vi "main.vi"() -> ()   [LabVIEW 2023]
panel:
  out "On/Off Light":bool
  in  "On/Off":bool
  out "Hours":i16
  out "Minutes":i16
  out "Seconds":i16
  in  "Stop":bool
  out "Waveform Chart - Temperatures":T1(graph)
  out "Waveform Chart - Control Signal":dbl[](graph)
  out "Temp [C]":dbl=29.659641078261295
  out "Error Term":dbl
  in  "Tab Control":T2(tab)=enum."Air heater model parameters"
  in  "Location of Sensor":string="Stue"
  out "Start seconds":dbl
  out "Logging seconds":dbl
  in  "MA Filter":bool=TRUE
  out "Control Signal [V]":dbl format="%#_2g"
  in  "Desired Temperature [deg C]":dbl(slide)=30.0 scale=20.0..40.0
  in  "Time Step [s]":dbl=0.1
  in  "Air Heater Params":T3={"Temp_init [C]"=22.0, "K [C/V]"=3.2, "theta_t [s]"=5.5, "theta_d [s]"=3.0, "theta_d_out_init [V]"=0.0, "theta_d_max [s]"=5.0}
  in  "Temp Environment [C]":dbl(slide)=22.0 scale=0.0..35.0
  # "Program Runtime:"
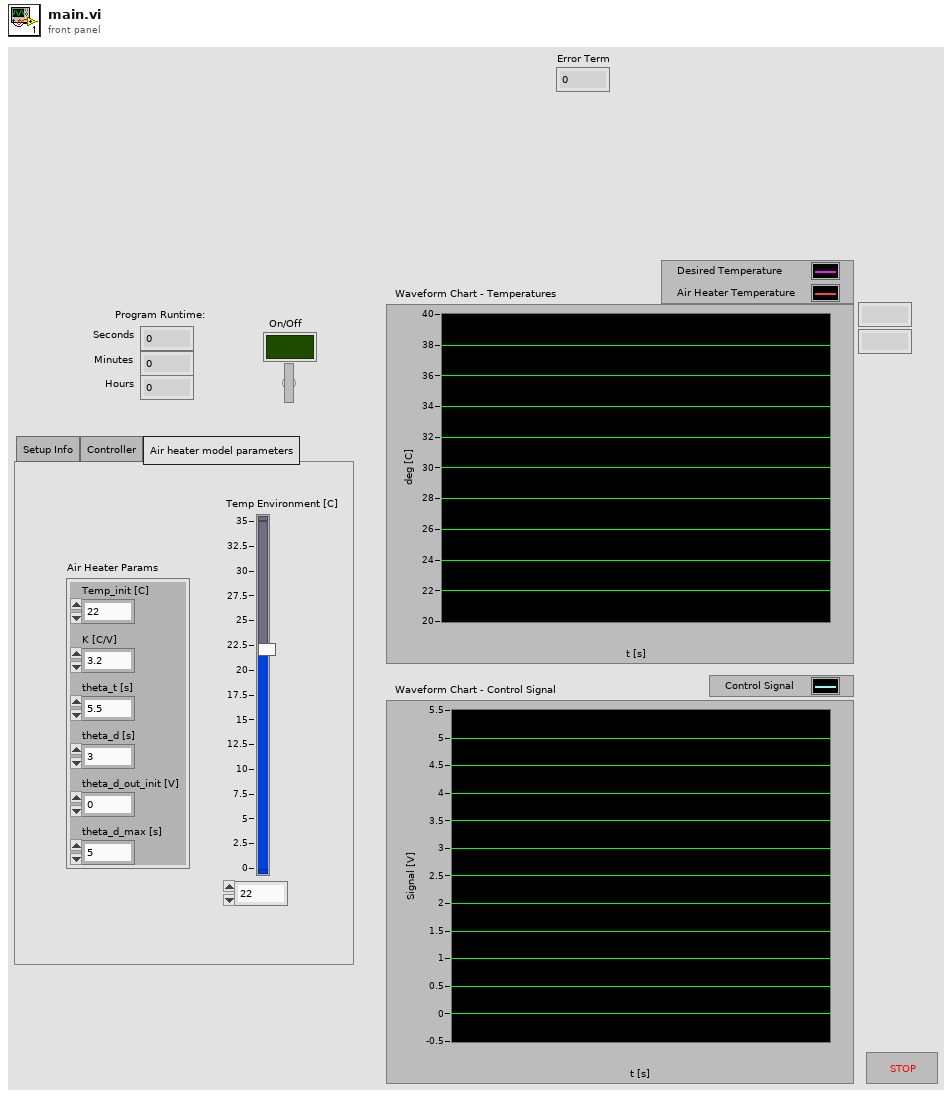
[diagram p1: front panel]
types:
  T1 = cluster{"Desired Temperature [deg C]":dbl, "Temp [C]":dbl}
  T2 = enum32{"Setup Info", "Controller", "Air heater model parameters"}
  T3 = cluster{"Temp_init [C]":dbl, "K [C/V]":dbl, "theta_t [s]":dbl, "theta_d [s]":dbl, "theta_d_out_init [V]":dbl, "theta_d_max [s]":dbl}
  T4 = cluster{"Desired Temperature [deg C]":dbl, "Temp [C]":dbl}[]
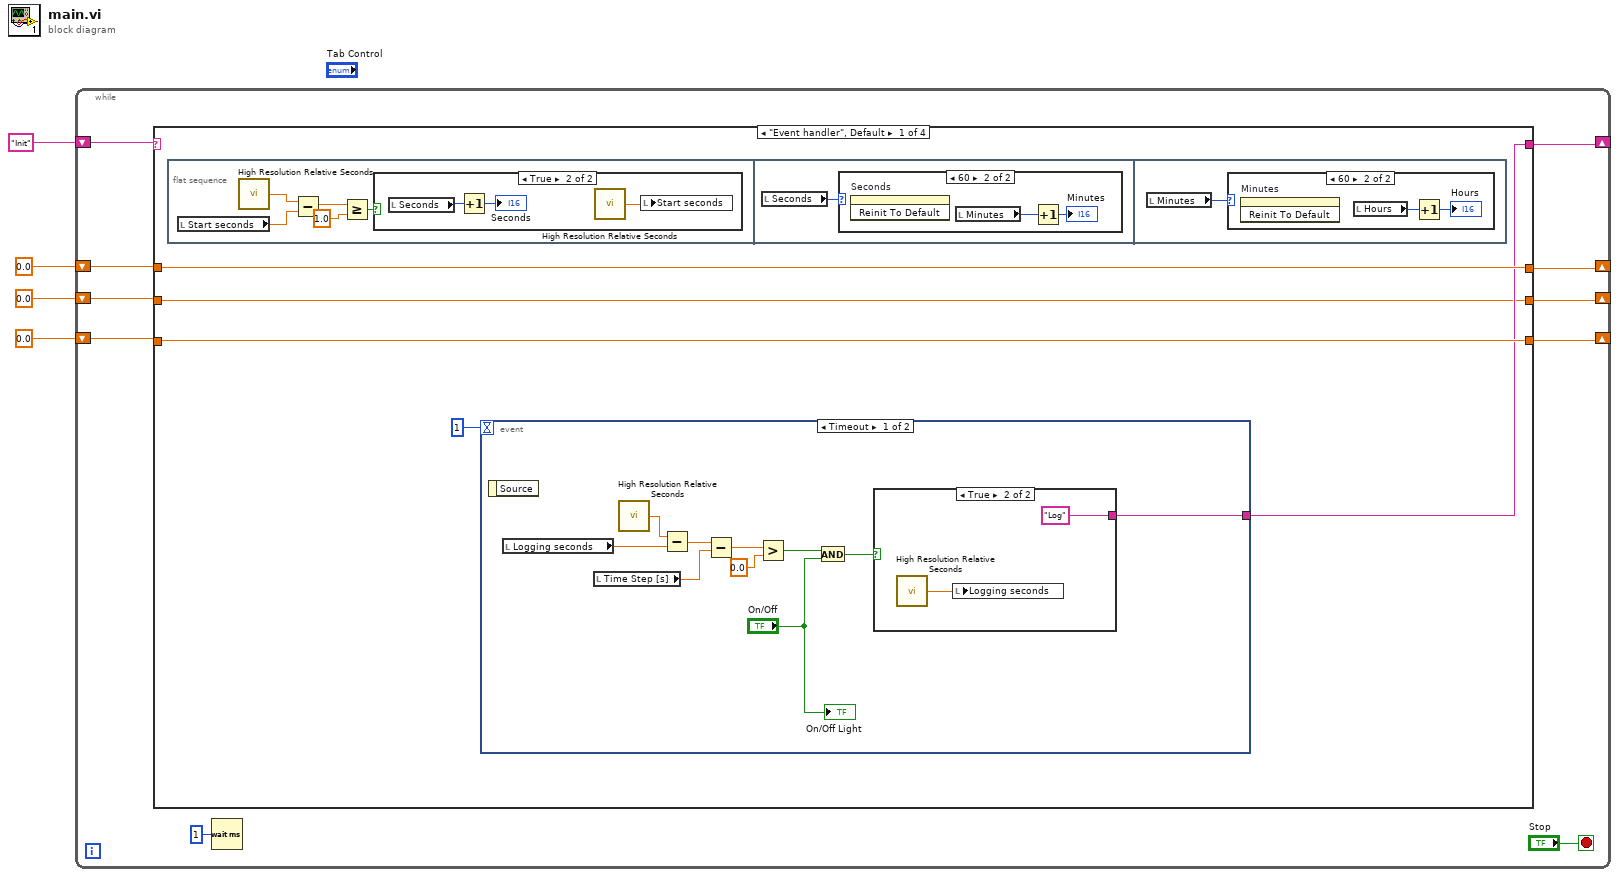
[diagram p0: block diagram]
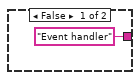
[diagram p2: hidden frame]
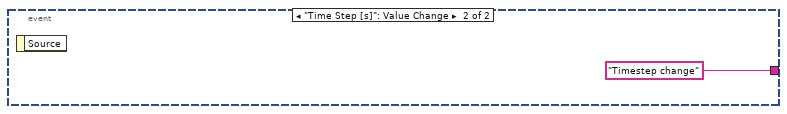
[diagram p3: hidden frame]
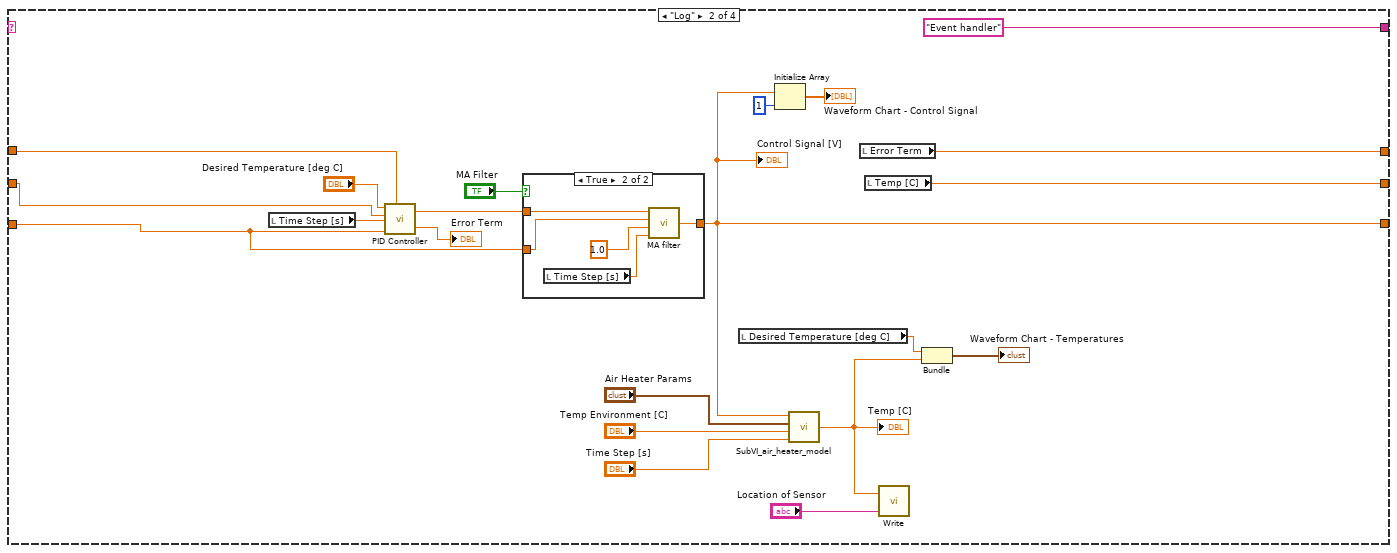
[diagram p7: hidden frame]
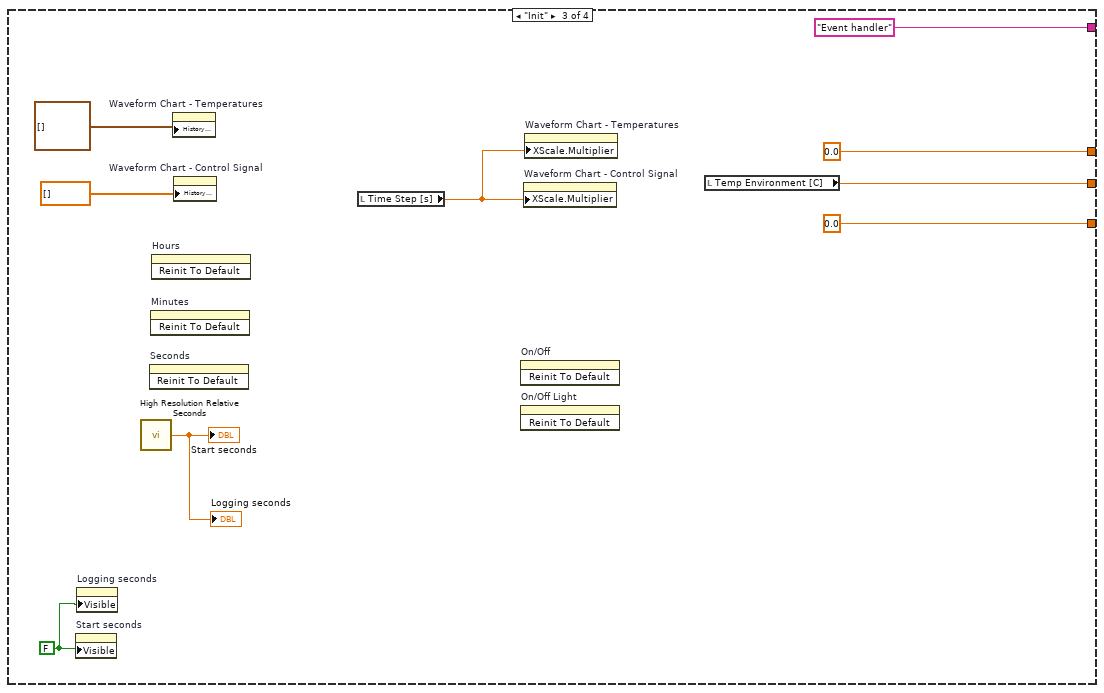
[diagram p9: hidden frame]
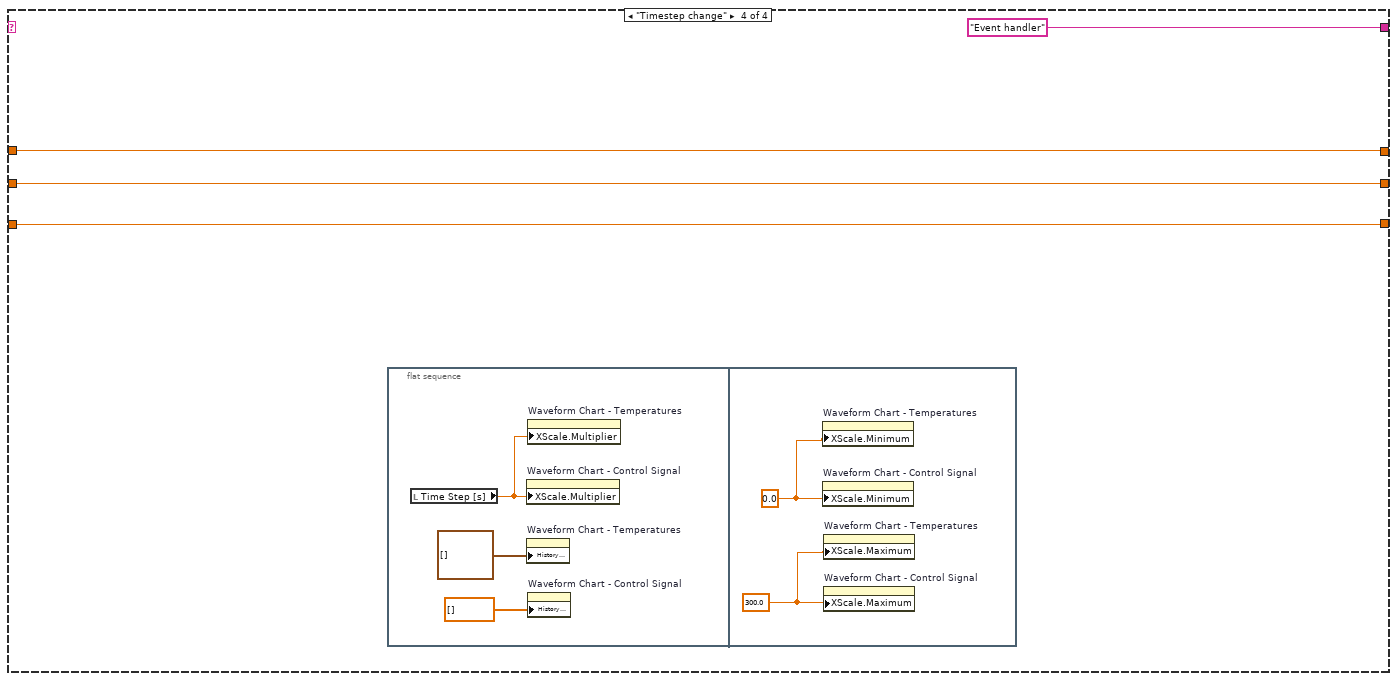
[diagram p10: hidden frame]
diagram:
  n1 = while {
    shift-right: [w8] -> _
    shift-left: "Init" -> [w13]
    shift-right: [w7] -> _
    shift-left: 0.0 ("yf") -> [w11]
    shift-right: [w6] -> _
    shift-left: 0.0 ("Error Term") -> [w10]
    shift-right: [w5] -> _
    shift-left: 0.0 ("Temp Environment [C]") -> [w9]
    stop <- "Stop" stop-if-true
    n2 = case shown="\"Event handler\", Default" w13 {
      tunnel: [w17 "Event handler" "Event handler" "Event handler"] -> w8
      tunnel: [w19 w52 0.0 ("yf") w87] -> w7
      tunnel: w11 -> [w19 w56 _ w87]
      tunnel: w10 -> [w18 w58 _ w86]
      tunnel: [w18 w57 0.0 ("Error Term") w86] -> w6
      tunnel: [w15 w55 w78 w84] -> w5
      tunnel: w9 -> [w15 w50 _ w84]
      frame "Event handler", Default {
        n3 = flat-sequence {
          frame #0 {
            n4 = local read "Start seconds"() -> (w37:dbl)
            n5 = call <vilib>:"High Resolution Relative Seconds.vi"() -> ("relative seconds"=w38:dbl)
            n6 = Subtract(x=w38, y=w37) -> (x-y=w36:dbl)
            n7 = Greater Or Equal?(x=w36, y=1.0) -> (x >= y?=w34:bool)
            n8 = case shown="True" w34 {
              frame False {
              }
              frame True {
                n9 = local read "Seconds"() -> (w39:i16)
                n10 = Increment(x=w39) -> (x+1=→"Seconds":i16)
                n11 = call <vilib>:"High Resolution Relative Seconds.vi"() -> ("relative seconds"=w41:dbl)
                n12 = local write "Start seconds"(w41) -> ()
              }
            }
          }
          frame #1 {
            n13 = local read "Seconds"() -> (w42:i16)
            n14 = case shown="60" w42 {
              frame 0, Default {
              }
              frame 60 {
                n15 = invoke on="Seconds" class="DigNum (strict)" method="Reinit To Default"() -> ()  [unwired: 3 in, 3 out]
                n16 = local read "Minutes"() -> (w43:i16)
                n17 = Increment(x=w43) -> (x+1=→"Minutes":i16)
              }
            }
          }
          frame #2 {
            n18 = local read "Minutes"() -> (w45:i16)
            n19 = case shown="60" w45 {
              frame 0, Default {
              }
              frame 60 {
                n20 = invoke on="Minutes" class="DigNum (strict)" method="Reinit To Default"() -> ()  [unwired: 3 in, 3 out]
                n21 = local read "Hours"() -> (w47:i16)
                n22 = Increment(x=w47) -> (x+1=→"Hours":i16)
              }
            }
          }
        }
        n23 = event shown="[0] Timeout" {
          selector: _ -> [_ _]
          dyn-events: _ -> [_ _]
          timeout: 1 -> [_ _]
          tunnel: [w25 "Timestep change"] -> w17
          event Timeout {
            n24 = event-data() -> ()  [unwired: 1 in, 1 out]
            n25 = local read "Logging seconds"() -> (w23:dbl)
            n26 = local read "Time Step [s]"() -> (w27:dbl)
            n27 = call <vilib>:"High Resolution Relative Seconds.vi"() -> ("relative seconds"=w29:dbl)
            n28 = Subtract(x=w29, y=w23) -> (x-y=w28:dbl)
            n29 = Subtract(x=w28, y=w27) -> (x-y=w24:dbl)
            n30 = Greater?(x=w24, y=0.0) -> (0:w21:bool)
            n31 = And(x=w21, y="On/Off") -> (x .and. y?=w20:bool)
            n32 = case shown="True" w20 {
              tunnel: ["Event handler" "Log"] -> w25
              frame False {
              }
              frame True {
                n33 = call <vilib>:"High Resolution Relative Seconds.vi"() -> ("relative seconds"=w31:dbl)
                n34 = local write "Logging seconds"(w31) -> ()
              }
            }
            "On/Off Light" <- "On/Off"
          }
          event "Time Step [s]": Value Change {
            n35 = event-data() -> ()  [unwired: 1 in, 1 out]
          }
        }
      }
      frame "Log" {
        n36 = local read "Time Step [s]"() -> (w65:dbl)
        n37 = call "PID Controller.vi"("Reference Value"="Desired Temperature [deg C]", "Process Value"=w50, "Time step [s]"=w65, "Previous signal"=w56, "Previous error"=w58) -> ("Process signal"=w67:dbl, "Error Term"=→"Error Term":dbl)
        n38 = case shown="True" "MA Filter" {
          tunnel: w67 -> [w69 w72]
          tunnel: [w69 w71] -> w52
          tunnel: w56 -> [_ w70]
          frame False {
          }
          frame True {
            n39 = local read "Time Step [s]"() -> (w74:dbl)
            n40 = call "MA filter.vi"("dt"=w74, "Tw"=1.0, "y_1"=w70, "y"=w72) -> ("yf"=w71:dbl)
          }
        }
        "Control Signal [V]" <- w52
        n41 = local read "Desired Temperature [deg C]"() -> (w62:dbl)
        n42 = Initialize Array(w52, 1 ("dimension size")) -> (→"Waveform Chart - Control Signal":dbl[])
        n43 = call "SubVI_air_heater_model.vi"("T_step [s]"="Time Step [s]", "Temp_env [C]"="Temp Environment [C]", "Cluster_air_heater_params"="Air Heater Params", "u [V]"=w52) -> ("Temp [C]"=w49:dbl)
        "Temp [C]" <- w49
        n44 = local read "Error Term"() -> (w57:dbl)
        n45 = local read "Temp [C]"() -> (w55:dbl)
        n46 = call "Write.vi"("Location of DAQ"="Location of Sensor", "Temperature from DAQ"=w49) -> ()  [unwired: 1 in]
        n47 = Bundle("Desired Temperature [deg C]"=w62, "Temp [C]"=w49) -> (→"Waveform Chart - Temperatures":T1)  [unwired: 1 in]
      }
      frame "Init" {
        w76 = FALSE ("Visible")
        n48 = property on="Start seconds" class="DigNum (strict)"("Visible"=w76) -> ()  [unwired: 2 in, 2 out]
        n49 = property on="Logging seconds" class="DigNum (strict)"("Visible"=w76) -> ()  [unwired: 2 in, 2 out]
        n50 = call <vilib>:"High Resolution Relative Seconds.vi"() -> ("relative seconds"=→"Start seconds" →"Logging seconds":dbl)
        n51 = invoke on="Seconds" class="DigNum (strict)" method="Reinit To Default"() -> ()  [unwired: 3 in, 3 out]
        n52 = invoke on="Minutes" class="DigNum (strict)" method="Reinit To Default"() -> ()  [unwired: 3 in, 3 out]
        n53 = invoke on="Hours" class="DigNum (strict)" method="Reinit To Default"() -> ()  [unwired: 3 in, 3 out]
        n54 = property on="Waveform Chart - Temperatures" class="WFChart (strict)"("History Data"=T4 []) -> ()  [unwired: 2 in, 2 out]
        n55 = property on="Waveform Chart - Control Signal" class="WFChart (strict)"("History Data"=dbl[] []) -> ()  [unwired: 2 in, 2 out]
        n56 = local read "Time Step [s]"() -> (w75:dbl)
        n57 = invoke on="On/Off" class="Bool (strict)" method="Reinit To Default"() -> ()  [unwired: 3 in, 3 out]
        n58 = invoke on="On/Off Light" class="Bool (strict)" method="Reinit To Default"() -> ()  [unwired: 3 in, 3 out]
        n59 = property on="Waveform Chart - Control Signal" class="WFChart (strict)"("XScale.Multiplier"=w75) -> ()  [unwired: 2 in, 2 out]
        n60 = property on="Waveform Chart - Temperatures" class="WFChart (strict)"("XScale.Multiplier"=w75) -> ()  [unwired: 2 in, 2 out]
        n61 = local read "Temp Environment [C]"() -> (w78:dbl)
      }
      frame "Timestep change" {
        n62 = flat-sequence {
          frame #0 {
            n63 = local read "Time Step [s]"() -> (w88:dbl)
            n64 = property on="Waveform Chart - Control Signal" class="WFChart (strict)"("XScale.Multiplier"=w88) -> ()  [unwired: 2 in, 2 out]
            n65 = property on="Waveform Chart - Temperatures" class="WFChart (strict)"("History Data"=T4 []) -> ()  [unwired: 2 in, 2 out]
            n66 = property on="Waveform Chart - Temperatures" class="WFChart (strict)"("XScale.Multiplier"=w88) -> ()  [unwired: 2 in, 2 out]
            n67 = property on="Waveform Chart - Control Signal" class="WFChart (strict)"("History Data"=dbl[] []) -> ()  [unwired: 2 in, 2 out]
          }
          frame #1 {
            w91 = 300.0 ("X Scale.Range:Maximum")
            w92 = 0.0 ("X Scale.Range:Minimum")
            n68 = property on="Waveform Chart - Temperatures" class="WFChart (strict)"("XScale.Minimum"=w92) -> ()  [unwired: 2 in, 2 out]
            n69 = property on="Waveform Chart - Control Signal" class="WFChart (strict)"("XScale.Minimum"=w92) -> ()  [unwired: 2 in, 2 out]
            n70 = property on="Waveform Chart - Temperatures" class="WFChart (strict)"("XScale.Maximum"=w91) -> ()  [unwired: 2 in, 2 out]
            n71 = property on="Waveform Chart - Control Signal" class="WFChart (strict)"("XScale.Maximum"=w91) -> ()  [unwired: 2 in, 2 out]
          }
        }
      }
    }
    n72 = Wait (ms)(milliseconds to wait=u32 1) -> ()  [unwired: 1 out]
  }
